vi "Avoid Obstacle.vi"(0 "Destination Longitude":dbl format="%#_9g", 1 "Destination Latitude":dbl format="%#_8g") -> ()   [LabVIEW 2011]
uses:
  _GlobalVariables&Libraries/ATV Program Global Variables.vi
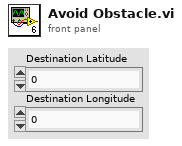
[diagram p1: front panel]
types:
  T1 = cluster{"GPS VISA resource name":refnum<visa-resource-name>, "GPS Error":errorcluster, "Disable GPS VISA":bool, "Latitude":dbl, "Longitude":dbl, "Latitude Uncertainty":dbl, "Longitude Uncertainty":dbl, "GPS Signal":u32}
  T2 = cluster{"Obstacle Detected":bool, "Drive Speed":string, "Steer Angle":string, "Left Object":bool, "Right Object":bool, "Center Object":bool, "Rear Left":bool, "Rear Right":bool}
  T3 = cluster{"End ATV Program":bool, "E-Stop":bool, "Save Logfile":bool, "Logfile Iteration Delay (ms)":u32, "Loop iteration time (ms)":u32, "Logfile Location":path, "Default GPS Navigation Path":path, "Computer":string, "Default GPS Boundary Path":path}
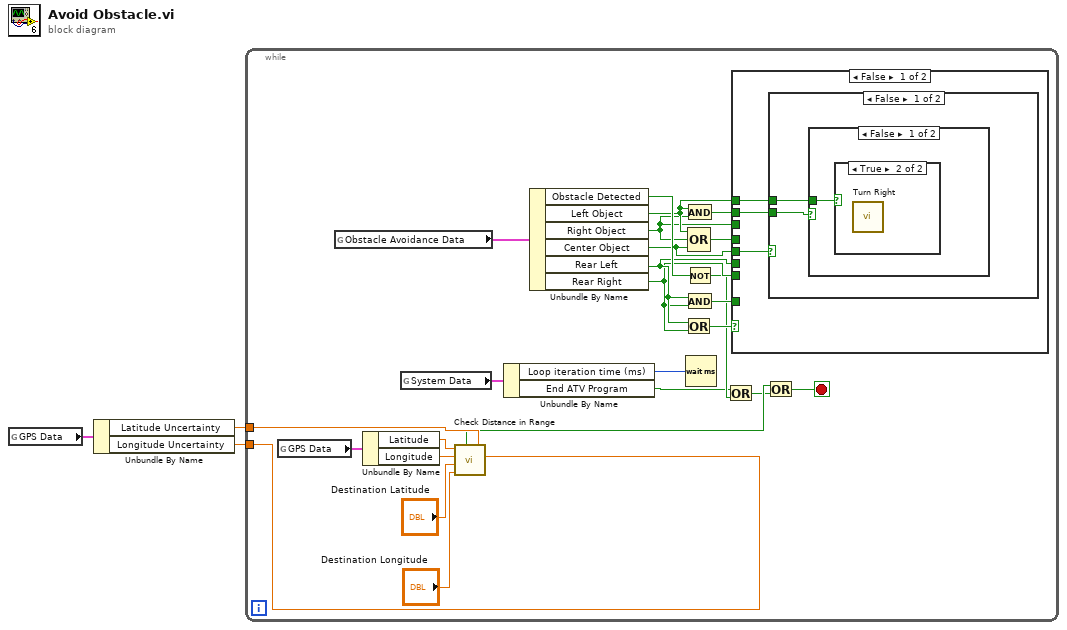
[diagram p0: block diagram]
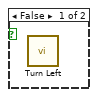
[diagram p2: hidden frame]
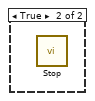
[diagram p3: hidden frame]
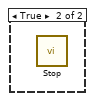
[diagram p4: hidden frame]
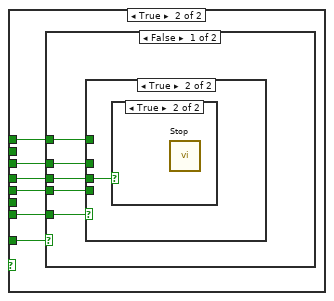
[diagram p5: hidden frame]
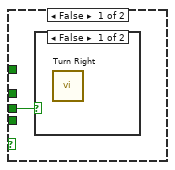
[diagram p6: hidden frame]
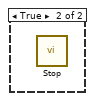
[diagram p7: hidden frame]
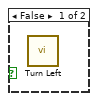
[diagram p8: hidden frame]
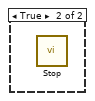
[diagram p9: hidden frame]
diagram:
  n1 = global read "ATV Program Global Variables.vi" "GPS Data"() -> (w3:T1)
  n2 = Unbundle By Name(w3) -> ("Latitude Uncertainty"=w2:dbl, "Longitude Uncertainty"=w1:dbl)
  n3 = while {
    tunnel: w2 -> [w10]
    tunnel: w1 -> [w9]
    stop <- w6 stop-if-true
    n4 = global read "ATV Program Global Variables.vi" "GPS Data"() -> (w13:T1)
    n5 = global read "ATV Program Global Variables.vi" "Obstacle Avoidance Data"() -> (w28:T2)
    n6 = Unbundle By Name(w13) -> ("Latitude"=w12:dbl, "Longitude"=w11:dbl)
    n7 = global read "ATV Program Global Variables.vi" "System Data"() -> (w26:T3)
    n8 = call "Check Distance in Range.vi"("Longitude Uncertainty"=w9, "Latitude Uncertainty"=w10, "Destination Longitude"="Destination Longitude", "Destination Latitude"="Destination Latitude", "Current Longitude"=w11, "Current Latitude"=w12) -> ("Distance in Range?"=w8:bool)  [unwired: 2 out]
    n9 = Unbundle By Name(w26) -> ("Loop iteration time (ms)"=w25:u32, "End ATV Program"=w14:bool)
    n10 = Unbundle By Name(w28) -> ("Obstacle Detected"=w27:bool, "Left Object"=w22:bool, "Right Object"=w21:bool, "Center Object"=w20:bool, "Rear Left"=w18:bool, "Rear Right"=w17:bool)
    n11 = Or(x=w18, y=w17) -> (x .or. y?=w24:bool)
    n12 = And(x=w22, y=w21) -> (x .and. y?=w23:bool)
    n13 = Not(x=w27) -> (.not. x?=w15:bool)
    n14 = And(x=w18, y=w17) -> (x .and. y?=w16:bool)
    n15 = Wait (ms)(milliseconds to wait=w25) -> ()  [unwired: 1 out]
    n16 = Compound Arithmetic op=OR(w22, w21, w20) -> (w19:bool)
    n17 = Or(x=w14, y=w15) -> (x .or. y?=w7:bool)
    n18 = case shown="False" w24 {
      tunnel: w18 -> [_ _]
      tunnel: w17 -> [_ w40]
      tunnel: w22 -> [w30 w39]
      tunnel: w20 -> [w29 w38]
      tunnel: w21 -> [_ w37]
      tunnel: w23 -> [w31 _]
      tunnel: w19 -> [_ w36]
      tunnel: w16 -> [_ w35]
      frame False {
        n19 = case shown="False" w29 {
          tunnel: w31 -> [w33 _]
          tunnel: w30 -> [w32 _]
          frame False {
            n20 = case shown="False" w33 {
              tunnel: w32 -> [w34 _]
              frame False {
                n21 = case shown="True" w34 {
                  frame False {
                    n22 = call "Turn Left.vi"() -> ()  [unwired: 12 in]
                  }
                  frame True {
                    n23 = call "Turn Right.vi"() -> ()  [unwired: 12 in]
                  }
                }
              }
              frame True {
                n24 = call "Stop.vi"() -> ()  [unwired: 12 in]
              }
            }
          }
          frame True {
            n25 = call "Stop.vi"() -> ()  [unwired: 12 in]
          }
        }
      }
      frame True {
        n26 = case shown="False" w35 {
          tunnel: w40 -> [w45 _]
          tunnel: w39 -> [w44 _]
          tunnel: w38 -> [w43 _]
          tunnel: w37 -> [w42 _]
          tunnel: w36 -> [w41 _]
          frame False {
            n27 = case shown="True" w45 {
              tunnel: w44 -> [_ _]
              tunnel: w43 -> [_ _]
              tunnel: w42 -> [_ _]
              tunnel: w41 -> [w46 w47]
              frame False {
                n28 = case shown="False" w46 {
                  frame False {
                    n29 = call "Turn Right.vi"() -> ()  [unwired: 12 in]
                  }
                  frame True {
                    n30 = call "Stop.vi"() -> ()  [unwired: 12 in]
                  }
                }
              }
              frame True {
                n31 = case shown="True" w47 {
                  frame False {
                    n32 = call "Turn Left.vi"() -> ()  [unwired: 12 in]
                  }
                  frame True {
                    n33 = call "Stop.vi"() -> ()  [unwired: 12 in]
                  }
                }
              }
            }
          }
          frame True {
            n34 = call "Stop.vi"() -> ()  [unwired: 12 in]
          }
        }
      }
    }
    n35 = Or(x=w8, y=w7) -> (x .or. y?=w6:bool)
  }
